vi "test io.vi"(1 "Call Context":T1) -> (0 "Test Data":T2)   [LabVIEW 2014]
uses:
  typedefs/test/test data.ctl
  <vilib>/Rock Robotics/WPI/DriverStation/WPI_DriverStationDerivedRobotMode.ctl
  global variables/safeties.vi
  global variables/devrefs.vi
panel:
  # "Get Test Data"
  # "Drive Encoders"
  # "Other Encoders"
  # "Safeties"
  # "Container Arm PID"
  # "Lift PID"
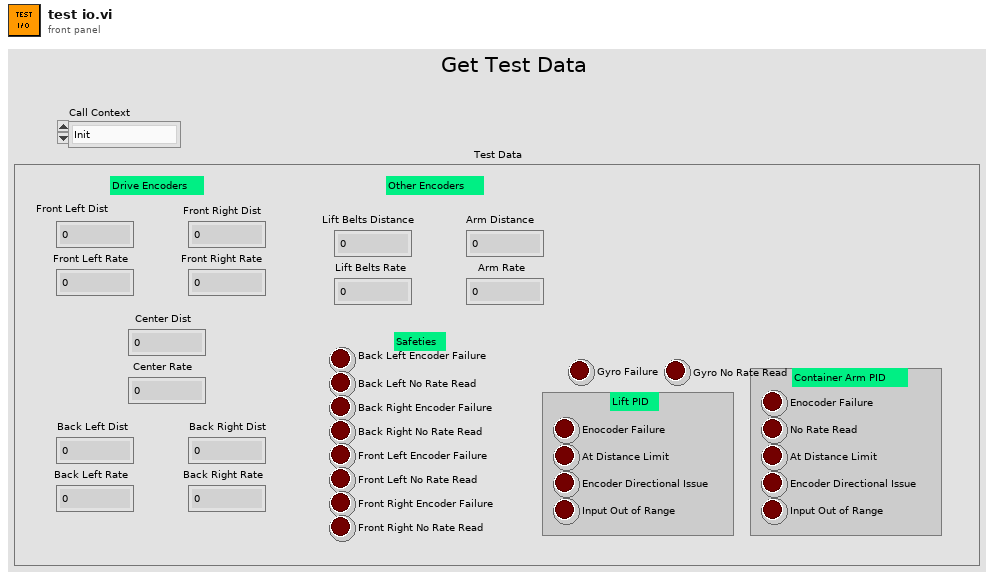
[diagram p1: front panel]
types:
  T1 = typedef "WPI_DriverStationDerivedRobotMode.ctl" = enum16{"Init", "Execute", "Stop"}
  T2 = typedef "test data.ctl" = cluster{"Back Left Encoder Failure":bool, "Front Left Dist":dbl, "Front Left Rate":dbl, "Front Right Dist":dbl, "Front Right Rate":dbl, "Center Dist":dbl, "Center Rate":dbl, "Back Left Dist":dbl, "Back Left Rate":dbl, "Back Right Dist":dbl, "Back Right Rate":dbl, "Lift Belts Distance":dbl, "Lift Belts Rate":dbl, "Arm Distance":dbl, "Arm Rate":dbl, "Back Left No Rate Read":bool, "Back Right Encoder Failure":bool, "Back Right No Rate Read":bool, "Front Left Encoder Failure":bool, "Front Left No Rate Read":bool, "Front Right Encoder Failure":bool, "Front Right No Rate Read":bool, "Enocoder Failure":bool, "At Distance Limit":bool, "Encoder Directional Issue":bool, "Input Out of Range":bool, "Enocoder Failure":bool, "No Rate Read":bool, "At Distance Limit":bool, "Encoder Directional Issue":bool, "Input Out of Range":bool, "Gyro Failure":bool, "Gyro No Rate Read":bool}
  T3 = typedef "WPI_EncoderDevRef.ctl" = cluster{"DevStatus":errorcluster, "EncoderIndex":T4, "CounterIndex":T5, "DistancePerCount":dbl, "Decoding Type":T6}
  T4 = typedef "FPGA_EncoderIdx.ctl" = enum8{"Enc 0", "Enc 1", "Enc 2", "Enc 3", "Enc 4", "Enc 5", "Enc 6", "Enc 7", "Invalid"}
  T5 = typedef "FPGA_CounterCtrSystemIndex.ctl" = enum8{"Ctr 0", "Ctr 1", "Ctr 2", "Ctr 3", "Ctr 4", "Ctr 5", "Ctr 6", "Ctr 7", "Invalid"}
  T6 = typedef "WPI_EncoderType.ctl" = enum16{"1x", "2x", "4x"}
  T7 = typedef "h-drive teleop safety data.ctl" = cluster{"Back Left Encoder Failure":bool, "Back Left No Rate Read":bool, "Back Right Encoder Failure":bool, "Back Right No Rate Read":bool, "Front Left Encoder Failure":bool, "Front Left No Rate Read":bool, "Front Right Encoder Failure":bool, "Front Right No Rate Read":bool, "No Gyro Rate Read":bool, "Gyro Failure":bool}
  T8 = typedef "container arm safety data.ctl" = cluster{"Encoder Disconnected":bool, "No Rate Read":bool, "At Distance Limit":bool, "Encoder Directional Issue":bool, "Input Out of Range":bool}
  T9 = typedef "lift safety data.ctl" = cluster{"Encoder Disconnected":bool, "At Distance Limit":bool, "Encoder Directional Issue":bool, "Input Out of Range":bool}
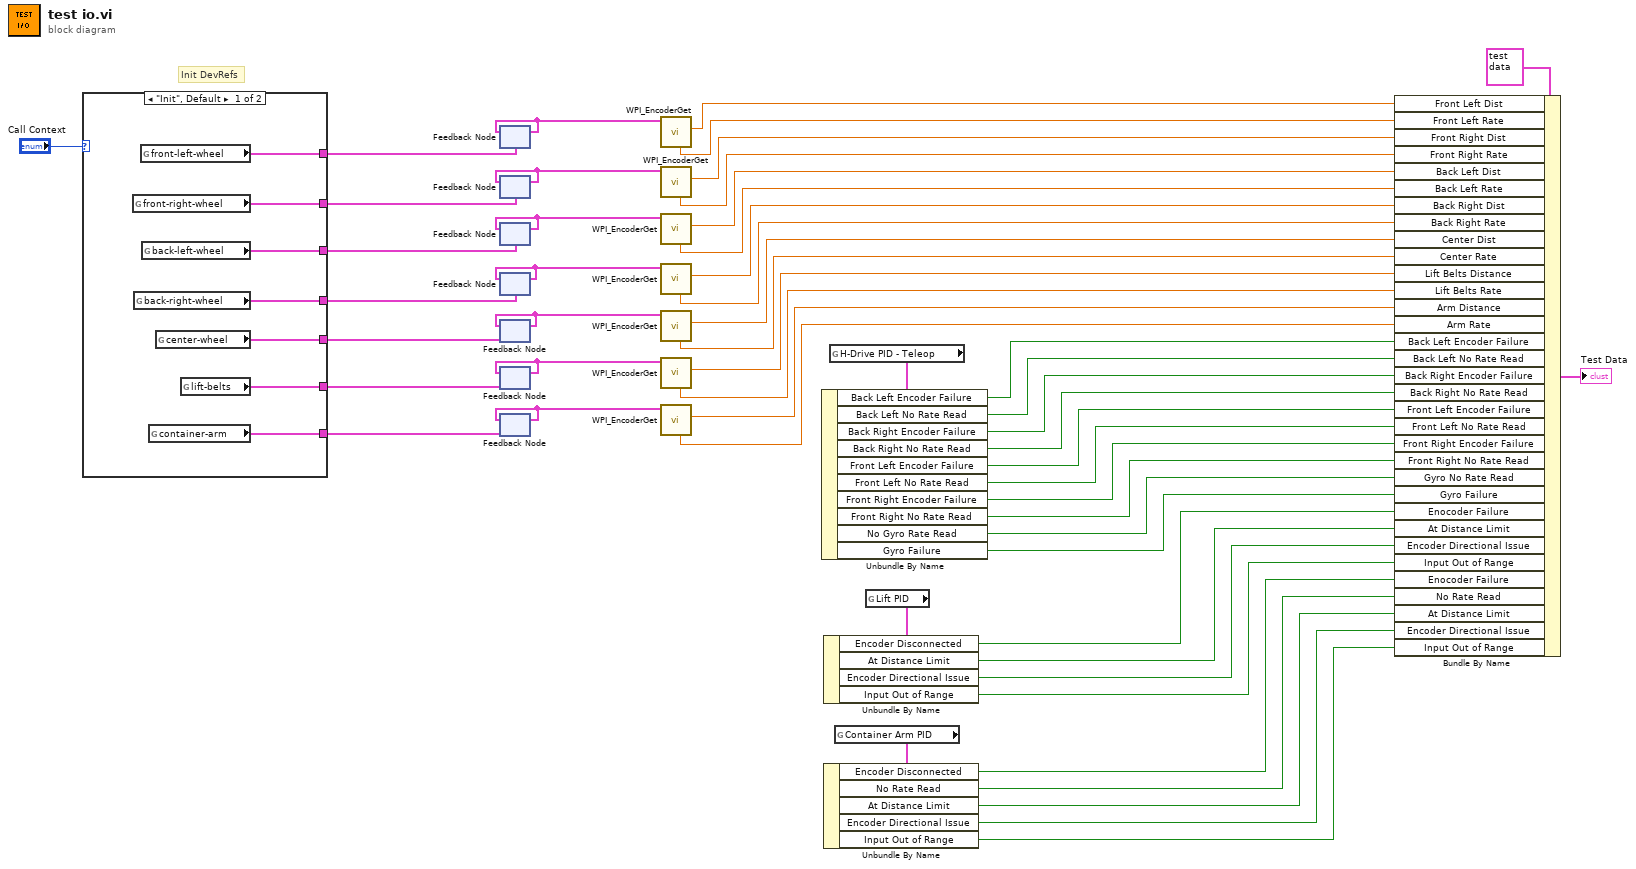
[diagram p0: block diagram]
diagram:
  # "Init DevRefs"
  n1 = case shown="\"Init\", Default" "Call Context" {
    tunnel: [w60 _] -> w52
    tunnel: [w59 _] -> w51
    tunnel: [w58 _] -> w49
    tunnel: [w57 _] -> w50
    tunnel: [w54 _] -> w38
    tunnel: [w55 _] -> w40
    tunnel: [w56 _] -> w39
    frame "Init", Default {
      n2 = global read "devrefs.vi" "front-right-wheel"() -> (w59:T3)
      n3 = global read "devrefs.vi" "back-right-wheel"() -> (w57:T3)
      n4 = global read "devrefs.vi" "front-left-wheel"() -> (w60:T3)
      n5 = global read "devrefs.vi" "back-left-wheel"() -> (w58:T3)
      n6 = global read "devrefs.vi" "container-arm"() -> (w56:T3)
      n7 = global read "devrefs.vi" "center-wheel"() -> (w54:T3)
      n8 = global read "devrefs.vi" "lift-belts"() -> (w55:T3)
    }
    frame "Execute", "Stop" {
      # "do nothing"
    }
  }
  n9 = feedback #1(w52) -> (w12:T3)
  n10 = feedback-in #1(w12) -> ()
  n11 = feedback #2(w51) -> (w11:T3)
  n12 = feedback-in #2(w11) -> ()
  n13 = feedback #3(w49) -> (w13:T3)
  n14 = feedback-in #3(w13) -> ()
  n15 = feedback #4(w50) -> (w14:T3)
  n16 = feedback-in #4(w14) -> ()
  n17 = feedback #5(w38) -> (w15:T3)
  n18 = feedback-in #5(w15) -> ()
  n19 = feedback #6(w40) -> (w16:T3)
  n20 = feedback-in #6(w16) -> ()
  n21 = feedback #7(w39) -> (w17:T3)
  n22 = feedback-in #7(w17) -> ()
  n23 = call <vilib>:"WPI_EncoderGet.vi"("EncoderDevRef"=w12) -> ("Distance"=w48:dbl, "Rate"=w47:dbl)  [unwired: 5 in, 4 out]
  n24 = call <vilib>:"WPI_EncoderGet.vi"("EncoderDevRef"=w11) -> ("Distance"=w46:dbl, "Rate"=w45:dbl)  [unwired: 5 in, 4 out]
  n25 = call <vilib>:"WPI_EncoderGet.vi"("EncoderDevRef"=w13) -> ("Distance"=w44:dbl, "Rate"=w43:dbl)  [unwired: 5 in, 4 out]
  n26 = call <vilib>:"WPI_EncoderGet.vi"("EncoderDevRef"=w14) -> ("Distance"=w42:dbl, "Rate"=w41:dbl)  [unwired: 5 in, 4 out]
  n27 = call <vilib>:"WPI_EncoderGet.vi"("EncoderDevRef"=w15) -> ("Distance"=w37:dbl, "Rate"=w36:dbl)  [unwired: 5 in, 4 out]
  n28 = call <vilib>:"WPI_EncoderGet.vi"("EncoderDevRef"=w16) -> ("Distance"=w35:dbl, "Rate"=w34:dbl)  [unwired: 5 in, 4 out]
  n29 = call <vilib>:"WPI_EncoderGet.vi"("EncoderDevRef"=w17) -> ("Distance"=w33:dbl, "Rate"=w32:dbl)  [unwired: 5 in, 4 out]
  n30 = global read "safeties.vi" "H-Drive PID - Teleop"() -> (w31:T7)
  n31 = Unbundle By Name(w31) -> ("Back Left Encoder Failure"=w30:bool, "Back Left No Rate Read"=w29:bool, "Back Right Encoder Failure"=w28:bool, "Back Right No Rate Read"=w27:bool, "Front Left Encoder Failure"=w26:bool, "Front Left No Rate Read"=w25:bool, "Front Right Encoder Failure"=w24:bool, "Front Right No Rate Read"=w23:bool, "No Gyro Rate Read"=w22:bool, "Gyro Failure"=w21:bool)
  n32 = global read "safeties.vi" "Container Arm PID"() -> (w19:T8)
  n33 = Unbundle By Name(w19) -> ("Encoder Disconnected"=w5:bool, "No Rate Read"=w4:bool, "At Distance Limit"=w3:bool, "Encoder Directional Issue"=w2:bool, "Input Out of Range"=w1:bool)
  n34 = global read "safeties.vi" "Lift PID"() -> (w20:T9)
  n35 = Unbundle By Name(w20) -> ("Encoder Disconnected"=w10:bool, "At Distance Limit"=w8:bool, "Encoder Directional Issue"=w7:bool, "Input Out of Range"=w6:bool)
  n36 = Bundle By Name(cluster=T2 {"Back Left Encoder Failure"=FALSE, "Front Left Dist"=0.0, "Front Left Rate"=0.0, "Front Right Dist"=0.0, "Front Right Rate"=0.0, "Center Dist"=0.0, "Center Rate"=0.0, "Back Left Dist"=0.0, "Back Left Rate"=0.0, "Back Right Dist"=0.0, "Back Right Rate"=0.0, "Lift Belts Distance"=0.0, "Lift Belts Rate"=0.0, "Arm Distance"=0.0, "Arm Rate"=0.0, "Back Left No Rate Read"=FALSE, "Back Right Encoder Failure"=FALSE, "Back Right No Rate Read"=FALSE, "Front Left Encoder Failure"=FALSE, "Front Left No Rate Read"=FALSE, "Front Right Encoder Failure"=FALSE, "Front Right No Rate Read"=FALSE, "Enocoder Failure"=FALSE, "At Distance Limit"=FALSE, "Encoder Directional Issue"=FALSE, "Input Out of Range"=FALSE, "Enocoder Failure"=FALSE, "No Rate Read"=FALSE, "At Distance Limit"=FALSE, "Encoder Directional Issue"=FALSE, "Input Out of Range"=FALSE, "Gyro Failure"=FALSE, "Gyro No Rate Read"=FALSE} ("Test Data"), "Front Left Dist"=w48, "Front Left Rate"=w47, "Front Right Dist"=w46, "Front Right Rate"=w45, "Back Left Dist"=w44, "Back Left Rate"=w43, "Back Right Dist"=w42, "Back Right Rate"=w41, "Center Dist"=w37, "Center Rate"=w36, "Lift Belts Distance"=w35, "Lift Belts Rate"=w34, "Arm Distance"=w33, "Arm Rate"=w32, "Back Left Encoder Failure"=w30, "Back Left No Rate Read"=w29, "Back Right Encoder Failure"=w28, "Back Right No Rate Read"=w27, "Front Left Encoder Failure"=w26, "Front Left No Rate Read"=w25, "Front Right Encoder Failure"=w24, "Front Right No Rate Read"=w23, "Gyro No Rate Read"=w22, "Gyro Failure"=w21, "Enocoder Failure"=w10, "At Distance Limit"=w8, "Encoder Directional Issue"=w7, "Input Out of Range"=w6, "Enocoder Failure"=w5, "No Rate Read"=w4, "At Distance Limit"=w3, "Encoder Directional Issue"=w2, "Input Out of Range"=w1) -> (→"Test Data":T2)
